vi "Calculate Days Effect.vi"(10 "array type (2D Dbl) in":u8[](array[numeric]), 11 "Number of days":i32) -> (2 "Population size":i32, 3 "array type (2D Dbl) out":u8[](array[numeric]))   [LabVIEW 2019, in "Day 6.lvlib"]
uses:
  Day 6.lvlib
panel:
  out "i":i32
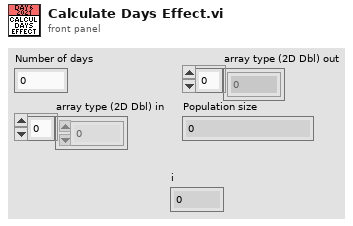
[diagram p1: front panel]
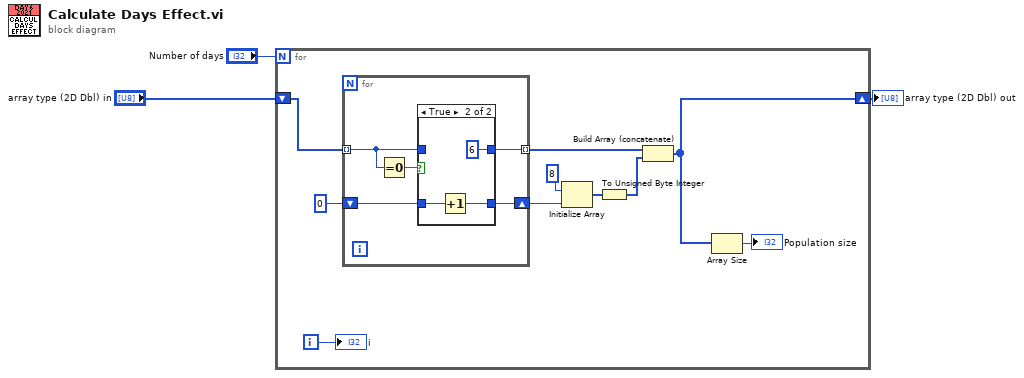
[diagram p0: block diagram]
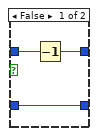
[diagram p2: hidden frame]
diagram:
  n1 = for {
    N: "Number of days" -> [_]
    shift-right: [w6] -> w1
    shift-left: "array type (2D Dbl) in" -> [w9]
    i -> [w5]
    n2 = for {
      tunnel: w9 -> [w17] mode=indexing
      tunnel: [w18] -> w10 mode=indexing
      shift-right: [w14] -> w11
      shift-left: u32 0 -> [w15]
      n3 = Equal To 0?(x=w17) -> (x = 0?=w16:bool)
      n4 = case shown="True" w16 {
        tunnel: [w21 u8 6] -> w18
        tunnel: w17 -> [w20 _]
        tunnel: w15 -> [w19 w23]
        tunnel: [w19 w22] -> w14
        frame False {
          n5 = Decrement(x=w20) -> (x-1=w21:u8)
        }
        frame True {
          n6 = Increment(x=w23) -> (x+1=w22:u32)
        }
      }
    }
    n7 = Initialize Array(u8 8, w11) -> (w7:u8[])
    n8 = To Unsigned Byte Integer(number=w7) -> (unsigned 8bit integer=w8:u8[])
    n9 = Build Array (concatenate)(w10, w8) -> (w6:u8[])
    n10 = Array Size(array=w6) -> (size(s)=→"Population size":i32)
    "i" <- w5
  }
  "array type (2D Dbl) out" <- w1
